vi "Kursovaya 3.vi"() -> ()   [LabVIEW 2013]
uses:
  <vilib>/measure/mascope.llb/Transition Measurements 1 chan.vi
  <vilib>/measure/mascope.llb/Pulse Measurements 1 chan.vi
  <vilib>/measure/NI_MAPro.lvlib
panel:
  in  "?":bool
  in  "?":bool
  out "?":dbl[](array[numeric])
  out "?":dbl[](array[numeric])
  out "?":dbl[](array[numeric])
  in  "?":bool
  in  "?":bool
  out "Вывод ошибки":string
  in  "?":bool
  in  "?":bool
  out "Длительность\nимпульса":dbl format="%.2g"
  out "Время \nподъёма":dbl
  out "?":bool
  out "Наличие \nсигнала":dbl
  out "Мак-ное\nзанчение":dbl
  in  "?":bool
  in  "VISA resource name":refnum<visa-resource-name>
  out "Экран осциллографаф":waveform(dbl)(graph)
  in  "Буфер":u32=15000
  in  "Канал (1: Channel 1)":u16(ring)=1 items=["Channel 1"=1, "Channel 2"=2, "Channel 3"=3, "Channel 4"=4]
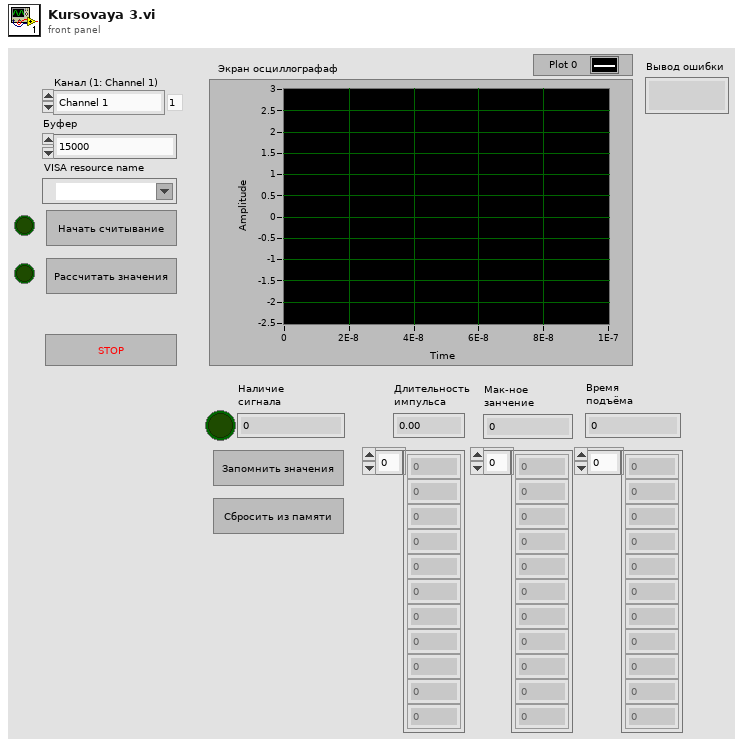
[diagram p1: front panel]
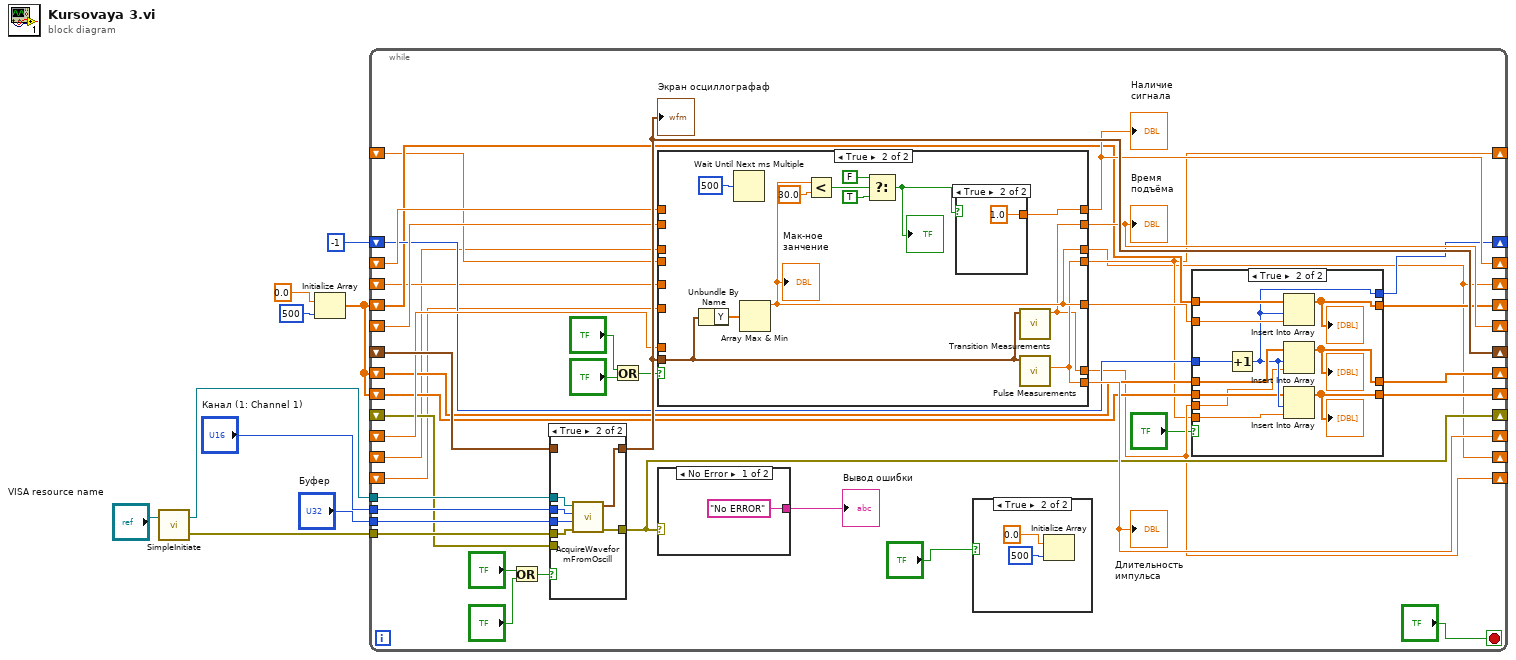
[diagram p0: block diagram]
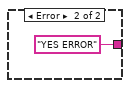
[diagram p4: hidden frame]
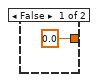
[diagram p6: hidden frame]
diagram:
  n1 = call "SimpleInitiate.vi"("VISA resource name"="VISA resource name") -> ("error out"=w9:errorcluster, "VISA resource name out"=w8:refnum<visa-resource-name>)  [unwired: 1 in]
  n2 = Initialize Array(0.0 ("element"), 500 ("dimension size")) -> (w1:dbl[])
  n3 = while {
    tunnel: w9 -> [w38]
    tunnel: w8 -> [w49]
    tunnel: "Канал (1: Channel 1)" -> [w48]
    tunnel: "Буфер" -> [w47]
    shift-right: [w46] -> _
    shift-left: _ -> [w45]
    shift-right: [w36] -> _
    shift-left: _ -> [w37]
    shift-right: [w44] -> _
    shift-left: _ -> [w43]
    shift-right: [w42] -> _
    shift-left: _ -> [w41]
    shift-right: [w40] -> _
    shift-left: _ -> [w39]
    shift-right: [w21] -> _
    shift-left: -1 -> [w27]
    shift-right: [w24] -> _
    shift-left: w1 -> [w25]
    shift-right: [w22] -> _
    shift-left: w1 -> [w23]
    shift-right: [w19] -> _
    shift-left: w1 -> [w20]
    shift-right: [w13] -> _
    shift-left: _ -> [w18]
    shift-right: [w17] -> _
    shift-left: _ -> [w16]
    shift-right: [w15] -> _
    shift-left: _ -> [w14]
    shift-right: [w13] -> _
    shift-left: _ -> [w12]
    stop <- "?" stop-if-true
    n4 = Or(x="?", y="?") -> (x .or. y?=w32:bool)
    n5 = case shown="True" w32 {
      tunnel: w49 -> [_ w97]
      tunnel: w48 -> [_ w96]
      tunnel: w47 -> [_ w95]
      tunnel: w38 -> [_ w94]
      tunnel: [w90 w93] -> w36
      tunnel: [w91 w92] -> w46
      tunnel: w45 -> [w91 _]
      tunnel: w37 -> [w90 _]
      frame False {
      }
      frame True {
        n6 = call "AcquireWaveformFromOscill.vi"("error in"=w94, "byte count"=w95, "Channel (1: Channel 1)"=w96, "VISA resource name"=w97) -> ("error out"=w93:errorcluster, "Waveform Graph"=w92:waveform(dbl))  [unwired: 2 out]
      }
    }
    "Экран осциллографаф" <- w46
    n7 = Or(x="?", y="?") -> (x .or. y?=w29:bool)
    n8 = case shown="True" w29 {
      tunnel: [w75 w82] -> w44
      tunnel: [w74 w76] -> w42
      tunnel: [w73 w77] -> w40
      tunnel: w46 -> [_ w81]
      tunnel: w43 -> [w75 _]
      tunnel: w41 -> [w74 _]
      tunnel: w39 -> [w73 _]
      tunnel: [w72 w78] -> w26
      tunnel: [w69 w78] -> w13
      tunnel: w18 -> [w72 _]
      tunnel: [w71 w76] -> w17
      tunnel: w16 -> [w71 _]
      tunnel: [w70 w77] -> w15
      tunnel: w14 -> [w70 _]
      tunnel: w12 -> [w69 _]
      frame False {
      }
      frame True {
        n9 = Unbundle By Name(w81) -> ("Y"=w80:dbl[])
        n10 = Wait Until Next ms Multiple(millisecond multiple=u32 500) -> ()  [unwired: 1 out]
        n11 = Array Max & Min(array=w80) -> (max value=w78:dbl)  [unwired: 3 out]
        "Мак-ное\nзанчение" <- w78
        n12 = Less?(x=w78, y=30.0) -> (x < y?=w86:bool)
        n13 = Select(t=FALSE, s=w86, f=TRUE) -> (s? t:f=w83:bool)
        "?" <- w83
        n14 = case shown="True" w83 {
          tunnel: [0.0 ("Numeric") 1.0 ("Numeric")] -> w82
          frame False {
          }
          frame True {
          }
        }
        n15 = call-poly <vilib>:"Transition Measurements.vi"("signal in"=w81) -> ("transition duration"=w76:dbl)  [unwired: 5 in, 5 out]
        n16 = call-poly <vilib>:"Pulse Measurements.vi"("signal in"=w81) -> ("pulse duration"=w77:dbl)  [unwired: 6 in, 4 out]
      }
    }
    "Наличие \nсигнала" <- w44
    "Время \nподъёма" <- w42
    "Длительность\nимпульса" <- w40
    n17 = case shown="No Error" w36 {
      tunnel: ["No ERROR" ("Error") "YES ERROR" ("Error")] -> w35
      frame No Error {
      }
      frame Error {
      }
    }
    "Вывод ошибки" <- w35
    n18 = case shown="True" "?" {
      frame False {
      }
      frame True {
        n19 = Initialize Array(0.0 ("element"), 500 ("dimension size")) -> ()  [unwired: 1 out]
      }
    }
    n20 = case shown="True" "?" {
      tunnel: w27 -> [w53 w66]
      tunnel: w26 -> [_ w65]
      tunnel: w25 -> [w55 w64]
      tunnel: [w55 w63] -> w24
      tunnel: w23 -> [w54 w62]
      tunnel: [w54 w61] -> w22
      tunnel: [w53 w60] -> w21
      tunnel: w20 -> [w52 w59]
      tunnel: [w52 w58] -> w19
      tunnel: w17 -> [_ w57]
      tunnel: w15 -> [_ w56]
      frame False {
      }
      frame True {
        n21 = Increment(x=w66) -> (x+1=w60:i32)
        n22 = Insert Into Array(array=w64, index=w60, new element=w65) -> (w63:dbl[])
        "?" <- w63
        n23 = Insert Into Array(array=w62, index=w60, new element=w57) -> (w61:dbl[])
        "?" <- w61
        n24 = Insert Into Array(array=w59, index=w60, new element=w56) -> (w58:dbl[])
        "?" <- w58
      }
    }
  }
